vi "Stop All Nested Actors.vi"(8 "error in (no error)":errorcluster, 10 "final error code":i32, 11 "Actor Nest in":refnum<class "Actor Nest.lvclass">) -> (0 "error out":errorcluster, 3 "Actor Nest out":refnum<class "Actor Nest.lvclass">)   [LabVIEW 2012, in "Actor Nest.lvlib" / "Actor Nest.lvclass"]
uses:
  Actor Nest.lvclass
  Actor Nest.lvclass/Actor Nest.ctl
  <vilib>/ActorFramework/Message Enqueuer/Message Enqueuer.lvclass
  <vilib>/ActorFramework/Stop Msg/Stop Msg.lvclass/Stop Msg.ctl
  <vilib>/ActorFramework/Message Enqueuer/Message Enqueuer.lvclass/Message Enqueuer.ctl
  <vilib>/ActorFramework/Stop Msg/Send Emergency Stop.vi
  <vilib>/ActorFramework/Stop Msg/Send Normal Stop.vi
  <vilib>/ActorFramework/Message Enqueuer/Enqueue Critical.vi
  <vilib>/ActorFramework/Message Enqueuer/Enqueue.vi
  <vilib>/ActorFramework/Message Priority Queue/Priority Enqueue.vi
  <vilib>/ActorFramework/Stop Msg/Stop Msg.lvclass
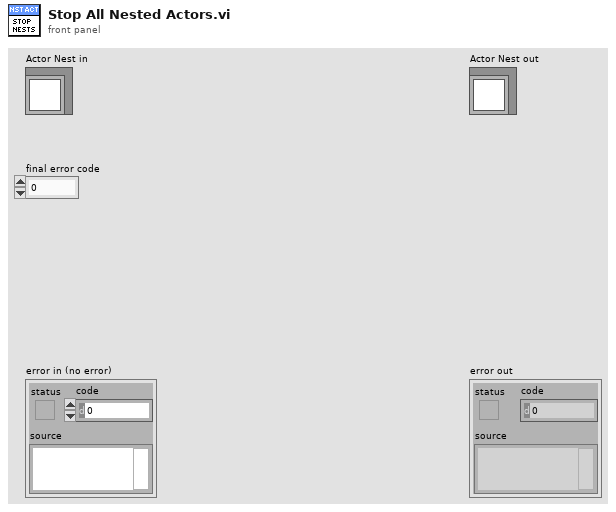
[diagram p1: front panel]
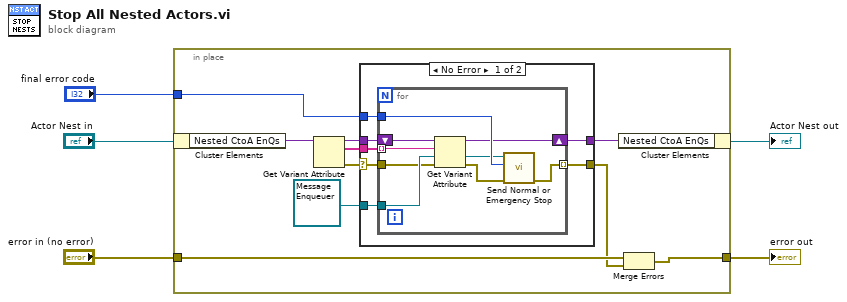
[diagram p0: block diagram]
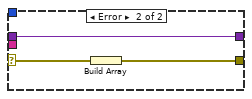
[diagram p2: hidden frame]
diagram:
  n1 = in-place {
    in-place-border: "final error code" -> [w10]
    in-place-border: "error in (no error)" -> [w9]
    in-place-border: [w7] -> w4
    n2 = in-place-cluster #1("Actor Nest in") -> ("Nested CtoA EnQs"=w12:variant)
    n3 = Get Variant Attribute(Variant=w12) -> (duplicate Variant=w13:variant, names=w14:string[], error out=w6:errorcluster)  [unwired: 3 in, 1 out]
    n4 = case shown="No Error" w6 {
      selector: w6 -> [w16 w33]
      tunnel: refnum<class "Message Enqueuer.lvclass"> refnum ("Message Enqueuer") -> [w22 _]
      tunnel: w14 -> [w21 _]
      tunnel: w13 -> [w20 w34]
      tunnel: [w19 w34] -> w11
      tunnel: w10 -> [w18 _]
      tunnel: [w17 w32] -> w8
      frame No Error {
        n5 = for {
          tunnel: w18 -> [w31]
          shift-right: [w26] -> w19
          shift-left: w20 -> [w30]
          tunnel: w21 -> [w29] mode=indexing
          tunnel: w22 -> [w28]
          tunnel: w16 -> [w25]
          tunnel: [w23] -> w17 mode=indexing
          n6 = Get Variant Attribute(Variant=w30, name=w29, default value (empty Variant)=w28, error in=w25) -> (duplicate Variant=w26:variant, value=w27:refnum<class "Message Enqueuer.lvclass">, error out=w24:errorcluster)  [unwired: 1 out]
          n7 = call <vilib>:"Send Normal or Emergency Stop.vi"("error in (no error)"=w24, "final error code"=w31, "Message Enqueuer"=w27) -> ("error out"=w23:errorcluster)  [unwired: 8 in]
        }
      }
      frame Error {
        n8 = Build Array(w33) -> (w32:errorcluster[])
      }
    }
    n9 = in-place-cluster #1("Nested CtoA EnQs"=w11) -> (→"Actor Nest out":refnum<class "Actor Nest.lvclass">)
    n10 = Merge Errors(w9, w8) -> (w7:errorcluster)
  }
  "error out" <- w4
